vi "VoltageChart.vi"() -> ()   [LabVIEW 2013]
uses:
  eng/trunk/ni/cRIO Master Files/Controls/StringSelector.ctl
panel:
  out "Voltage Difference":sgl
  out "Waveform Chart":T1(graph)
  in  "stop":bool
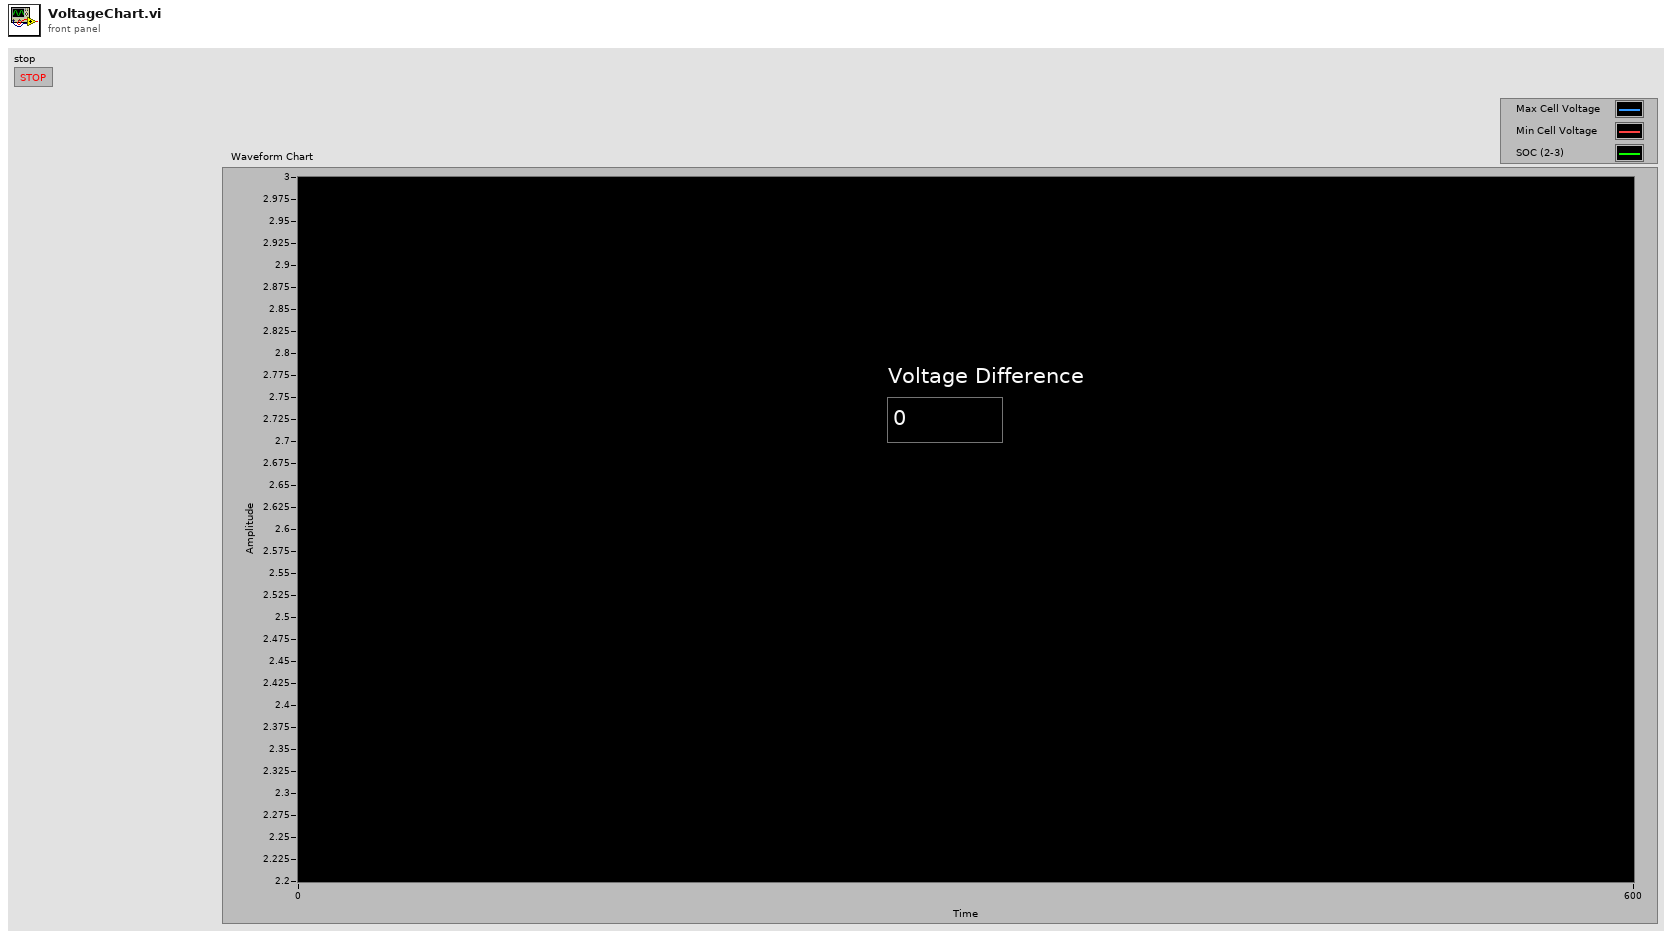
[diagram p1: front panel]
types:
  T1 = cluster{"[0]":sgl, "[1]":sgl, "[2]":sgl, "[3]":sgl, "[4]":sgl, "[5]":sgl, "[6]":sgl, "[7]":sgl, "[8]":sgl}
  T2 = typedef "StringSelector.ctl" = enum16{"1 String (1)", "1 String (2)", "1 String (3)", "2 Strings (1, 2)", "2 Strings (2, 3)", "2 Strings (1, 3)", "3 Strings"}
  T3 = cluster{"Voltage":sgl, "Current":sgl, "SOC Avg":sgl, "Faults":u16, "Alarms":u16, "Number of Strings":u16, "Max Temp":i16, "Min Temp":i16, "Max Cell Voltage":sgl, "Min Cell Voltage":sgl, "Energy Capacity (kWh)":sgl, "Energy Remaining (kWh)":sgl, "SOC Min":sgl, "SOC Max":sgl, "ES Fault":bool, "String Selector":T2}
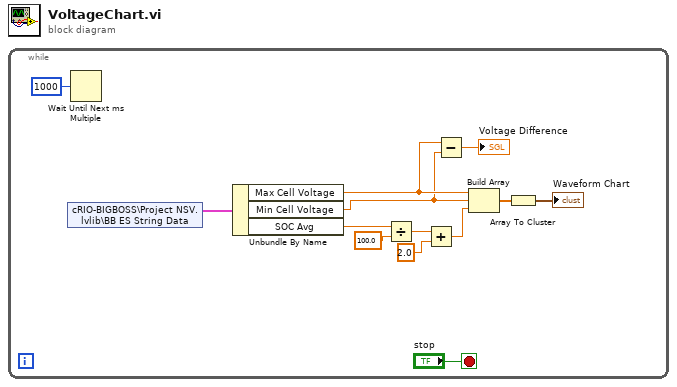
[diagram p0: block diagram]
diagram:
  n1 = while {
    stop <- "stop" stop-if-true
    n2 = shared-variable "cRIO-BIGBOSS\\Project NSV.lvlib\\BB ES String Data"() -> (w11:T3)  [unwired: 1 in, 1 out]
    n3 = Wait Until Next ms Multiple(millisecond multiple=u32 1000) -> ()  [unwired: 1 out]
    n4 = Unbundle By Name(w11) -> ("Max Cell Voltage"=w3:sgl, "Min Cell Voltage"=w2:sgl, "SOC Avg"=w10:sgl)
    n5 = Divide(x=w10, y=sgl 100.0) -> (x/y=w8:sgl)
    n6 = Add(x=w8, y=sgl 2.0) -> (x+y=w6:sgl)
    n7 = Subtract(x=w3, y=w2) -> (x-y=→"Voltage Difference":sgl)
    n8 = Build Array(w3, w2, w6) -> (w5:sgl[])
    n9 = Array To Cluster(array=w5) -> (cluster=→"Waveform Chart":T1)
  }
